vi "SimLIDARPlot.vi"(1 "data array [mag, phase (deg)]":cluster{"magnitude":dbl, "phase":dbl}[](array[cluster])) -> (0 "SONAR":picture)   [LabVIEW 2012]
doc: "This SubVI creates a polar plot of the incomming sonar data"
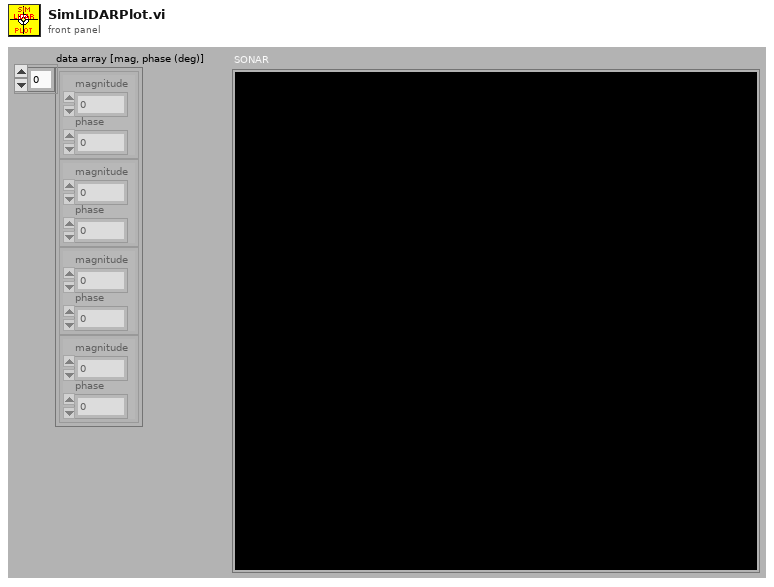
[diagram p1: front panel]
types:
  T1 = cluster{"Width":u16, "Style":enum32{"Solid", "Dash", "Dot", "DashDot", "DashDotDot"}}
  T2 = cluster{"maximum":dbl, "minimum":dbl, "clip to min":bool, "log?(F)":bool, "grid color":u32, "plot color":u32, "fmt and prec":cluster{"format":enum8{"Decimal", "Scientific", "Engineering", "Binary", "Octal", "Hex"}, "precision":u8}, "visible section":u16}
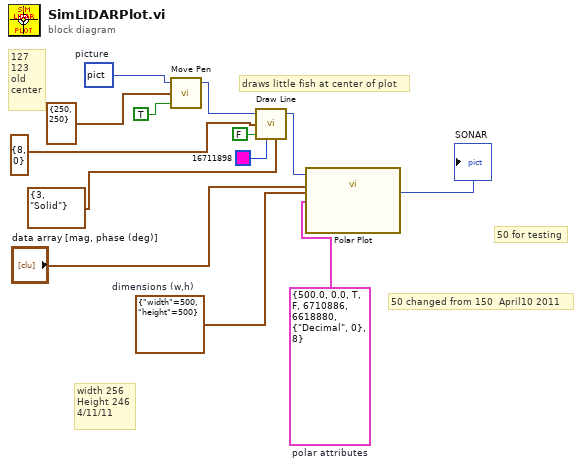
[diagram p0: block diagram]
diagram:
  w11 = cluster{"width":i16, "height":i16} {"width"=500, "height"=500}  # dimensions (w,h)
  w9 = picture data[5B]  # picture
  w13 = T2 {"maximum"=500.0, "minimum"=0.0, "clip to min"=TRUE, "log?(F)"=FALSE, "grid color"=6710886, "plot color"=6618880, "fmt and prec"={"format"=enum."Decimal", "precision"=0}, "visible section"=8}  # polar attributes
  # "127\n123\nold\ncenter"
  # "width 256\nHeight 246\n4/11/11"
  # "50 changed from 150  April10 2011"
  # "draws little fish at center of plot"
  # "50 for testing"
  n1 = call <vilib>:"Move Pen.vi"("absolute coordinates?(T)"=TRUE, "new position"=cluster{"x":i16, "y":i16} {"x"=250, "y"=250} ("point(x,y)"), "picture"=w9) -> ("new picture"=w10:picture)  [unwired: 2 in]
  n2 = call <vilib>:"Draw Line.vi"("picture"=w10, "end point"=cluster{"x":i16, "y":i16} {"x"=8, "y"=0}, "absolute coordinates?(T)"=FALSE, "color(black)"=u32 16711898, "pen"=T1 {"Width"=3, "Style"=enum."Solid"}) -> ("new picture"=w6:picture)  [unwired: 4 in]
  n3 = call <vilib>:"Polar Plot.vi"("polar attributes"=w13, "dimensions (w,h)"=w11, "data array [mag, phase (deg)]"="data array [mag, phase (deg)]", "picture"=w6) -> ("new picture"=→"SONAR":picture)  [unwired: 7 in]
